vi "all plate position.vi"(3 "position 15ml":T2={"X(A1)"=102.0, "Y(A1)"=332.0, "X(B1) "=266.0, "Y(B6) "=365.0, "count X"=6, "count Y"=2}, 4 "position 30ml":T2={"X(A1)"=102.0, "Y(A1)"=165.0, "X(B1) "=266.0, "Y(B6) "=200.0, "count X"=6, "count Y"=2}, 5 "position 2ml":T1={"X(A1)"=122.0, "Y(A1)"=124.0, "X(F9) "=226.0, "Y(F9) "=60.0, "count X"=9, "count Y"=6}) -> (0 "position3":dbl[][](array[numeric]), 1 "position2":dbl[][](array[numeric]), 2 "position1":dbl[][](array[numeric]))   [LabVIEW 2023]
uses:
  Shared variables/position1.vi
  Shared variables/position2.vi
  Shared variables/position3.vi
  Shared variables/Shared variables.lvlib
panel:
  in  "Tab Control":enum32{"2ml", "30ml", "15ml"}(tab)
  out "delta X":dbl
  out "delta Y":dbl
  out "total":i32
  out "Array X":dbl[](array[numeric])
  out "Array Y":dbl[](array[numeric])
  out "delta X 2":dbl
  out "Array X 2":dbl[](array[numeric])
  out "Array Y 2":dbl[](array[numeric])
  out "delta Y 2":dbl
  out "total 2":i32
  out "delta X 3":dbl
  out "Array X 3":dbl[](array[numeric])
  out "Array Y 3":dbl[](array[numeric])
  out "delta Y 3":dbl
  out "total 3":i32
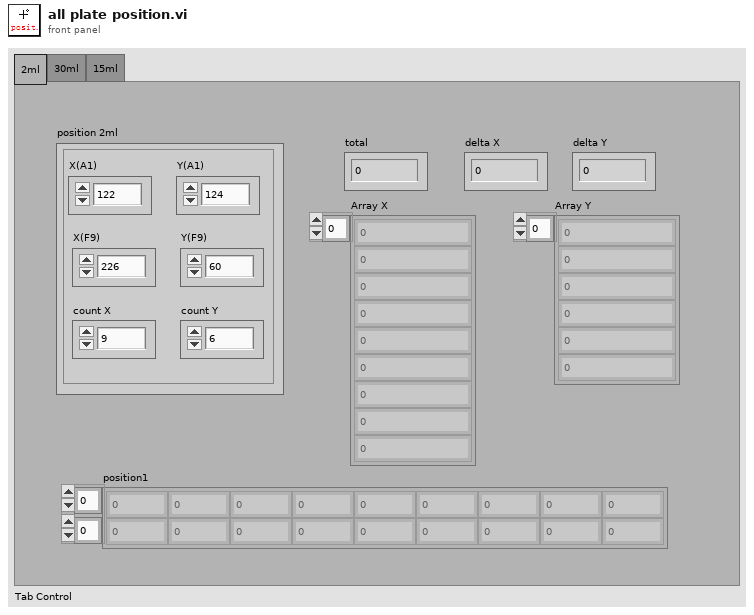
[diagram p1: front panel]
types:
  T1 = cluster{"X(A1)":dbl, "Y(A1)":dbl, "X(F9) ":dbl, "Y(F9) ":dbl, "count X":i32, "count Y":i32}
  T2 = cluster{"X(A1)":dbl, "Y(A1)":dbl, "X(B1) ":dbl, "Y(B6) ":dbl, "count X":i32, "count Y":i32}
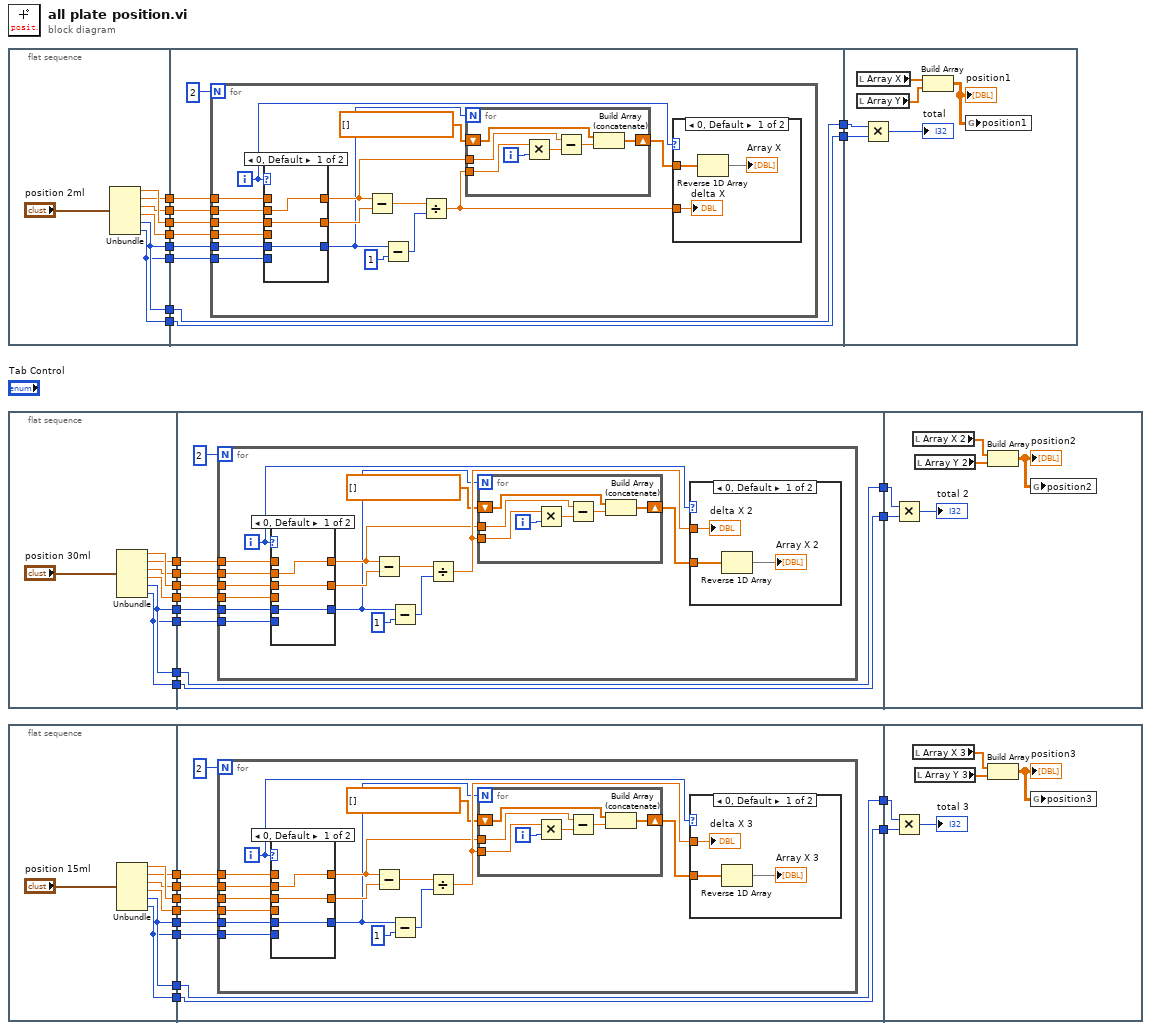
[diagram p0: block diagram]
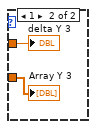
[diagram p2: hidden frame]
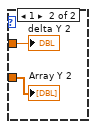
[diagram p4: hidden frame]
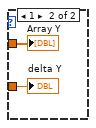
[diagram p6: hidden frame]
diagram:
  n1 = flat-sequence {
    tunnel: [w37] -> w30
    tunnel: [w36] -> w29
    tunnel: [w35] -> w28
    tunnel: [w34] -> w27
    tunnel: [w33] -> w26
    tunnel: [w32] -> w25
    tunnel: [w33] -> w23
    tunnel: [w32] -> w21
    tunnel: w30 -> [w45]
    tunnel: w29 -> [w44]
    tunnel: w28 -> [w43]
    tunnel: w27 -> [w42]
    tunnel: w26 -> [w41]
    tunnel: w25 -> [w40]
    tunnel: [w39] -> w24
    tunnel: w23 -> [w39]
    tunnel: [w38] -> w22
    tunnel: w21 -> [w38]
    tunnel: w24 -> [w85]
    tunnel: w22 -> [w84]
    frame #0 {
      n2 = Unbundle("position 2ml") -> ("X(A1)"=w37:dbl, "Y(A1)"=w36:dbl, "X(F9)"=w35:dbl, "Y(F9)"=w34:dbl, "count X"=w33:i32, "count Y"=w32:i32)
    }
    frame #1 {
      n3 = for {
        N: 2 -> [_]
        tunnel: w45 -> [w52]
        tunnel: w44 -> [w51]
        tunnel: w43 -> [w50]
        tunnel: w42 -> [w49]
        tunnel: w41 -> [w48]
        tunnel: w40 -> [w47]
        i -> [w54]
        n4 = case shown="0, Default" w54 {
          tunnel: w51 -> [_ w73]
          tunnel: w49 -> [_ w72]
          tunnel: w52 -> [w69 _]
          tunnel: w50 -> [w70 _]
          tunnel: [w70 w73] -> w56
          tunnel: [w69 w72] -> w55
          tunnel: [w68 w71] -> w53
          tunnel: w47 -> [_ w71]
          tunnel: w48 -> [w68 _]
          frame 0, Default {
          }
          frame 1 {
          }
        }
        n5 = Subtract(x=w56, y=w55) -> (x-y=w59:dbl)
        n6 = Subtract(x=w53, y=1) -> (x-y=w57:i32)
        n7 = Divide(x=w59, y=w57) -> (x/y=w62:dbl)
        n8 = for {
          N: w53 -> [_]
          shift-right: [w74] -> w61
          shift-left: dbl[] [] -> [w80]
          tunnel: w56 -> [w79]
          tunnel: w62 -> [w77]
          i -> [w78]
          n9 = Multiply(x=w77, y=w78) -> (x*y=w76:dbl)
          n10 = Subtract(x=w79, y=w76) -> (x-y=w75:dbl)
          n11 = Build Array (concatenate)(w80, w75) -> (w74:dbl[])
        }
        n12 = case shown="0, Default" w54 {
          tunnel: w62 -> [w65 w67]
          tunnel: w61 -> [w64 w66]
          frame 0, Default {
            n13 = Reverse 1D Array(array=w64) -> (reversed array=→"Array X":dbl[])
            "delta X" <- w65
          }
          frame 1 {
            "delta Y" <- w67
            "Array Y" <- w66
          }
        }
      }
    }
    frame #2 {
      n14 = local read "Array X"() -> (w83:dbl[])
      n15 = local read "Array Y"() -> (w82:dbl[])
      n16 = Multiply(x=w85, y=w84) -> (x*y=→"total":i32)
      n17 = Build Array(w83, w82) -> (w81:dbl[][])
      "position1" <- w81
      n18 = global write "position1.vi" "position1"(w81) -> ()
    }
  }
  n19 = flat-sequence {
    tunnel: [w92] -> w20
    tunnel: [w91] -> w19
    tunnel: [w90] -> w18
    tunnel: [w89] -> w17
    tunnel: [w88] -> w16
    tunnel: [w87] -> w15
    tunnel: [w88] -> w14
    tunnel: [w87] -> w13
    tunnel: w20 -> [w101]
    tunnel: w19 -> [w100]
    tunnel: w18 -> [w99]
    tunnel: w17 -> [w98]
    tunnel: w16 -> [w97]
    tunnel: w15 -> [w96]
    tunnel: [w95] -> w12
    tunnel: w14 -> [w95]
    tunnel: [w94] -> w11
    tunnel: w13 -> [w94]
    tunnel: w12 -> [w141]
    tunnel: w11 -> [w140]
    frame #0 {
      n20 = Unbundle("position 30ml") -> ("X(A1)"=w92:dbl, "Y(A1)"=w91:dbl, "X(B1)"=w90:dbl, "Y(B6)"=w89:dbl, "count X"=w88:i32, "count Y"=w87:i32)
    }
    frame #1 {
      n21 = for {
        N: 2 -> [_]
        tunnel: w101 -> [w108]
        tunnel: w100 -> [w107]
        tunnel: w99 -> [w106]
        tunnel: w98 -> [w105]
        tunnel: w97 -> [w104]
        tunnel: w96 -> [w103]
        i -> [w110]
        n22 = case shown="0, Default" w110 {
          tunnel: w107 -> [_ w129]
          tunnel: w105 -> [_ w128]
          tunnel: w108 -> [w125 _]
          tunnel: w106 -> [w126 _]
          tunnel: [w126 w129] -> w112
          tunnel: [w125 w128] -> w111
          tunnel: [w124 w127] -> w109
          tunnel: w103 -> [_ w127]
          tunnel: w104 -> [w124 _]
          frame 0, Default {
          }
          frame 1 {
          }
        }
        n23 = Subtract(x=w112, y=w111) -> (x-y=w115:dbl)
        n24 = Subtract(x=w109, y=1) -> (x-y=w113:i32)
        n25 = Divide(x=w115, y=w113) -> (x/y=w118:dbl)
        n26 = for {
          N: w109 -> [_]
          shift-right: [w130] -> w117
          shift-left: dbl[] [] -> [w136]
          tunnel: w112 -> [w135]
          tunnel: w118 -> [w133]
          i -> [w134]
          n27 = Multiply(x=w133, y=w134) -> (x*y=w132:dbl)
          n28 = Subtract(x=w135, y=w132) -> (x-y=w131:dbl)
          n29 = Build Array (concatenate)(w136, w131) -> (w130:dbl[])
        }
        n30 = case shown="0, Default" w110 {
          tunnel: w118 -> [w121 w123]
          tunnel: w117 -> [w120 w122]
          frame 0, Default {
            n31 = Reverse 1D Array(array=w120) -> (reversed array=→"Array X 2":dbl[])
            "delta X 2" <- w121
          }
          frame 1 {
            "delta Y 2" <- w123
            "Array Y 2" <- w122
          }
        }
      }
    }
    frame #2 {
      n32 = Multiply(x=w141, y=w140) -> (x*y=→"total 2":i32)
      n33 = local read "Array X 2"() -> (w139:dbl[])
      n34 = local read "Array Y 2"() -> (w138:dbl[])
      n35 = Build Array(w139, w138) -> (w137:dbl[][])
      "position2" <- w137
      n36 = global write "position2.vi" "position2"(w137) -> ()
    }
  }
  n37 = flat-sequence {
    tunnel: [w148] -> w10
    tunnel: [w147] -> w9
    tunnel: [w146] -> w8
    tunnel: [w145] -> w7
    tunnel: [w144] -> w6
    tunnel: [w143] -> w5
    tunnel: [w144] -> w4
    tunnel: [w143] -> w3
    tunnel: w10 -> [w157]
    tunnel: w9 -> [w156]
    tunnel: w8 -> [w155]
    tunnel: w7 -> [w154]
    tunnel: w6 -> [w153]
    tunnel: w5 -> [w152]
    tunnel: [w151] -> w2
    tunnel: w4 -> [w151]
    tunnel: [w150] -> w1
    tunnel: w3 -> [w150]
    tunnel: w2 -> [w197]
    tunnel: w1 -> [w196]
    frame #0 {
      n38 = Unbundle("position 15ml") -> ("X(A1)"=w148:dbl, "Y(A1)"=w147:dbl, "X(B1)"=w146:dbl, "Y(B6)"=w145:dbl, "count X"=w144:i32, "count Y"=w143:i32)
    }
    frame #1 {
      n39 = for {
        N: 2 -> [_]
        tunnel: w157 -> [w164]
        tunnel: w156 -> [w163]
        tunnel: w155 -> [w162]
        tunnel: w154 -> [w161]
        tunnel: w153 -> [w160]
        tunnel: w152 -> [w159]
        i -> [w166]
        n40 = case shown="0, Default" w166 {
          tunnel: w163 -> [_ w185]
          tunnel: w161 -> [_ w184]
          tunnel: w164 -> [w181 _]
          tunnel: w162 -> [w182 _]
          tunnel: [w182 w185] -> w168
          tunnel: [w181 w184] -> w167
          tunnel: [w180 w183] -> w165
          tunnel: w159 -> [_ w183]
          tunnel: w160 -> [w180 _]
          frame 0, Default {
          }
          frame 1 {
          }
        }
        n41 = Subtract(x=w168, y=w167) -> (x-y=w171:dbl)
        n42 = Subtract(x=w165, y=1) -> (x-y=w169:i32)
        n43 = Divide(x=w171, y=w169) -> (x/y=w174:dbl)
        n44 = for {
          N: w165 -> [_]
          shift-right: [w186] -> w173
          shift-left: dbl[] [] -> [w192]
          tunnel: w168 -> [w191]
          tunnel: w174 -> [w189]
          i -> [w190]
          n45 = Multiply(x=w189, y=w190) -> (x*y=w188:dbl)
          n46 = Subtract(x=w191, y=w188) -> (x-y=w187:dbl)
          n47 = Build Array (concatenate)(w192, w187) -> (w186:dbl[])
        }
        n48 = case shown="0, Default" w166 {
          tunnel: w174 -> [w177 w179]
          tunnel: w173 -> [w176 w178]
          frame 0, Default {
            n49 = Reverse 1D Array(array=w176) -> (reversed array=→"Array X 3":dbl[])
            "delta X 3" <- w177
          }
          frame 1 {
            "delta Y 3" <- w179
            "Array Y 3" <- w178
          }
        }
      }
    }
    frame #2 {
      n50 = Multiply(x=w197, y=w196) -> (x*y=→"total 3":i32)
      n51 = local read "Array X 3"() -> (w195:dbl[])
      n52 = local read "Array Y 3"() -> (w194:dbl[])
      n53 = Build Array(w195, w194) -> (w193:dbl[][])
      "position3" <- w193
      n54 = global write "position3.vi" "position3"(w193) -> ()
    }
  }
